vi "Right Click Menu Selected.vi"(8 "error in (no error)":errorcluster, 9 "Panel":string, 10 "Tag":string, 11 "SubPanel User Interface in":refnum<class "SubPanel User Interface.lvclass">) -> (0 "error out":errorcluster, 3 "SubPanel User Interface out":refnum<class "SubPanel User Interface.lvclass">)   [LabVIEW 2019, in "SubPanel User Interface.lvlib" / "SubPanel User Interface.lvclass"]
uses:
  SubPanel User Interface.lvclass
  SubPanel User Interface.lvclass/SubPanel User Interface.ctl
  UI Reference Wrapper/UI Reference Wrapper.lvclass/UI Reference Wrapper.ctl
  UI Reference Wrapper/Read VI Reference.vi
  UI Reference Wrapper/Write VI Reference.vi
  UI Reference Wrapper/UI Reference Wrapper.lvclass
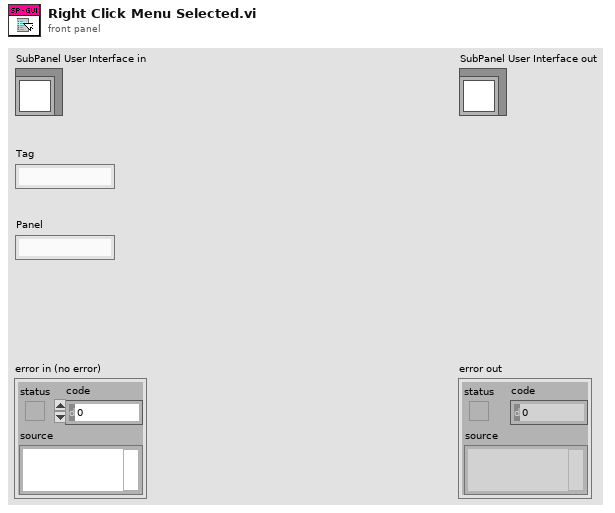
[diagram p1: front panel]
types:
  T1 = enum32{"Invalid", "Standard", "Closed", "Hidden", "Minimized", "Maximized"}
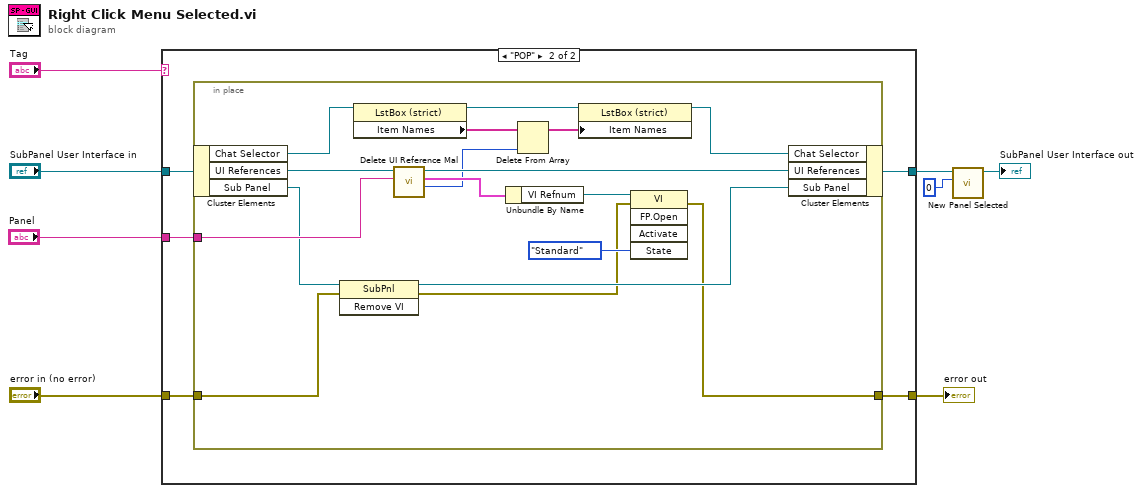
[diagram p0: block diagram]
diagram:
  n1 = case shown="\"POP\"" "Tag" {
    tunnel: "SubPanel User Interface in" -> [w10 w11]
    tunnel: "error in (no error)" -> [w9 w15]
    tunnel: [w10 w14] -> w3
    tunnel: [w9 w12] -> w5
    tunnel: "Panel" -> [_ w13]
    frame "False", Default {
    }
    frame "POP" {
      n2 = in-place {
        in-place-border: w15 -> [w17]
        in-place-border: w13 -> [w21]
        in-place-border: [w16] -> w12
        n3 = in-place-cluster #1(w11) -> ("Chat Selector"=w28:refnum<vi>, "UI References"=w25:refnum<class "UI Reference Wrapper.lvclass">, "Sub Panel"=w19:refnum<vi>)
        n4 = invoke class="SubPnl" method="Remove VI"(reference=w19, error in=w17) -> (reference out=w26:refnum<vi>, error out=w18:errorcluster)  [unwired: 1 in, 1 out]
        n5 = property class="LstBox (strict)"(reference=w28) -> (reference out=w31:refnum<vi>, "Item Names"=w30:string[])  [unwired: 1 in, 1 out]
        n6 = call "Delete UI Reference Mal.vi"("Panel"=w21, "UI Reference Wrapper in"=w25) -> ("Index"=w20:i32, "deleted portion"=w23:cluster{"VI Refnum":refnum<vi>, "Name":string}, "UI Reference Wrapper out"=w24:refnum<class "UI Reference Wrapper.lvclass">)  [unwired: 6 in, 1 out]
        n7 = Unbundle By Name(w23) -> ("VI Refnum"=w22:refnum<vi>)
        n8 = Delete From Array(array=w30, index=w20) -> (array with subset deleted=w29:string[])  [unwired: 1 in, 1 out]
        n9 = property class="LstBox (strict)"(reference=w31, "Item Names"=w29) -> (reference out=w27:refnum<vi>)  [unwired: 1 in, 1 out]
        n10 = invoke class="VI" method="FP.Open"(reference=w22, error in=w18, "State"=T1."Standard") -> (error out=w16:errorcluster)  [unwired: 2 in, 4 out]
        n11 = in-place-cluster #1("Chat Selector"=w27, "UI References"=w24, "Sub Panel"=w26) -> (w14:refnum<class "SubPanel User Interface.lvclass">)
      }
    }
  }
  "error out" <- w5
  n12 = call "New Panel Selected.vi"("Chat Window"=0, "SubPanel User Interface in"=w3) -> ("SubPanel User Interface out"=→"SubPanel User Interface out":refnum<class "SubPanel User Interface.lvclass">)  [unwired: 8 in, 1 out]
